vi "tmp_checked_wip.vi"() -> ()   [LabVIEW 2014]
panel:
  in  "Correction":dbl
  out "Current Speed":dbl
  in  "Encoder Value":dbl
  in  "Change/update":dbl
  in  "MS/update":u32
  in  "Desired Speed":dbl
  # "Always have DS divisible by C/u!"
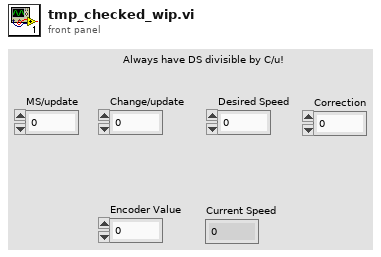
[diagram p1: front panel]
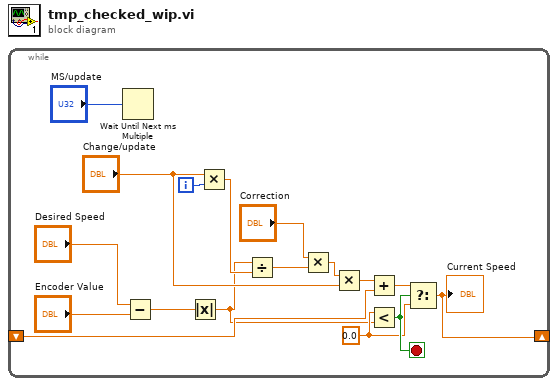
[diagram p0: block diagram]
diagram:
  n1 = while {
    shift-right: [w10] -> _
    shift-left: _ -> [w9]
    i -> [w4]
    stop <- w14 stop-if-true
    w12 = 0.0 ("f")
    n2 = Wait Until Next ms Multiple(millisecond multiple="MS/update") -> ()  [unwired: 1 out]
    n3 = Subtract(x="Desired Speed", y="Encoder Value") -> (x-y=w15:dbl)
    n4 = Absolute Value(x=w15) -> (abs(x)=w2:dbl)
    n5 = Multiply(x="Change/update", y=w4) -> (x*y=w5:dbl)
    n6 = Divide(x=w2, y=w5) -> (x/y=w1:dbl)
    n7 = Multiply(x="Correction", y=w1) -> (x*y=w6:dbl)
    n8 = Multiply(x=w6, y="Change/update") -> (x*y=w7:dbl)
    n9 = Add(x=w7, y=w9) -> (x+y=w11:dbl)
    n10 = Less?(x=w12, y=w2) -> (x < y?=w14:bool)
    n11 = Select(t=w11, s=w14, f=w12) -> (s? t:f=w10:dbl)
    "Current Speed" <- w10
  }
